vi "4.2 Surface Area and Volume of a Sphere-Prob1.vi"() -> ()   [LabVIEW 2025]
panel:
  out "Surface":dbl
  out "Volume":dbl
  in  "d":dbl
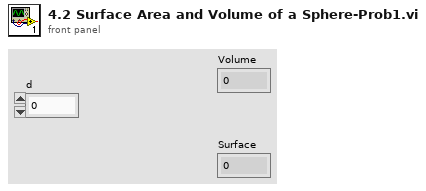
[diagram p1: front panel]
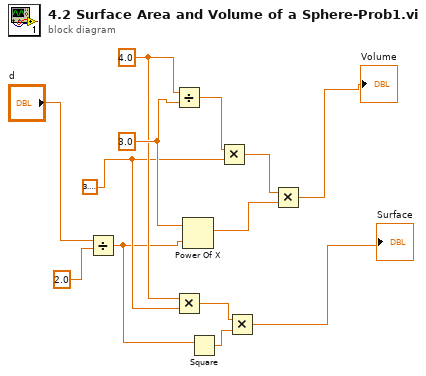
[diagram p0: block diagram]
diagram:
  w5 = 3.141592653589793
  w10 = 3.0
  w6 = 4.0
  n1 = Divide(x="d", y=2.0) -> (x/y=w2:dbl)
  n2 = Divide(x=w6, y=w10) -> (x/y=w13:dbl)
  n3 = Multiply(x=w6, y=w5) -> (x*y=w3:dbl)
  n4 = Power Of X(1:w2, 2:w10) -> (0:w9:dbl)
  n5 = Square(x=w2) -> (x^2=w4:dbl)
  n6 = Multiply(x=w13, y=w5) -> (x*y=w8:dbl)
  n7 = Multiply(x=w3, y=w4) -> (x*y=→"Surface":dbl)
  n8 = Multiply(x=w8, y=w9) -> (x*y=→"Volume":dbl)
